vi "Init DAQ.vi"(8 "error in":errorcluster, 11 "Notifiers in":T1) -> (0 "error out":errorcluster, 3 "Notifiers out":T1)   [LabVIEW 2014, in "DAQ.lvlib"]
uses:
  DAQ.lvlib
  support/Message Queue/Message Queue.lvlib
  Support/Message Queue/Enqueue Message (Single).vi
  PLC/PLC.lvlib
  Support/Notifiers/Notifiers.ctl
  Support/Notifiers/Notifiers.lvlib
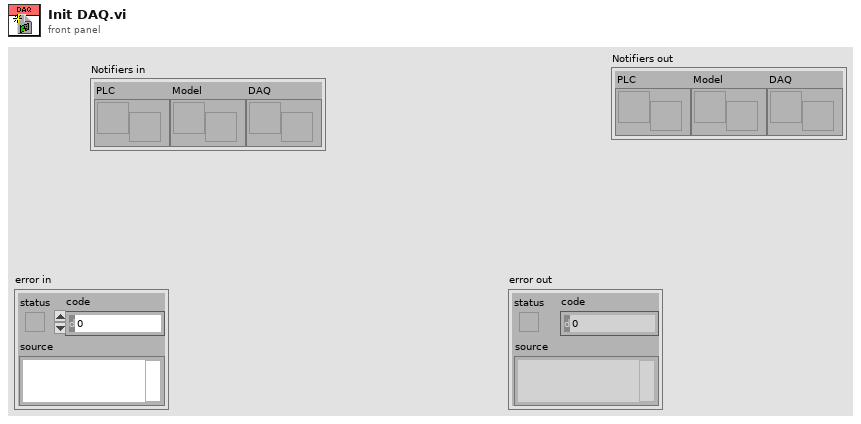
[diagram p1: front panel]
types:
  T1 = typedef "Notifiers.lvlib/Notifiers.ctl" = cluster{"PLC":refnum<notifier>, "Model":refnum<notifier>, "DAQ":refnum<notifier>}
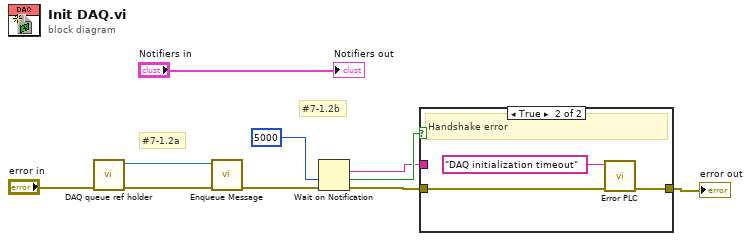
[diagram p0: block diagram]
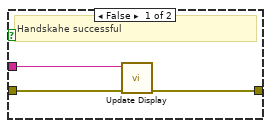
[diagram p2: hidden frame]
diagram:
  # "#7-1.2b"
  # "#7-1.2a"
  n1 = call "DAQ queue ref holder.vi"("error in"="error in") -> ("error out"=w3:errorcluster, "Input Message Queue"=w2:refnum<queue>)  [unwired: 9 in]
  n2 = call-poly "Enqueue Message.vi"("error in (no error)"=w3, "Message Queue"=w2) -> ("error out"=w6:errorcluster)  [unwired: 8 in, 1 out]
  n3 = Wait on Notification(timeout in ms (-1)=5000, error in (no error)=w6) -> (notification=w5:string, timed out?=w8:bool, error out=w9:errorcluster)  [unwired: 2 in, 1 out]
  n4 = case shown="True" w8 {
    tunnel: w9 -> [w12 w15]
    tunnel: [w11 w14] -> w10
    tunnel: w5 -> [w13 _]
    frame False {
      # "Handskahe successful"
      n5 = call "Update Display.vi"("error in"=w12, "Message string"=w13) -> ("error out"=w11:errorcluster)  [unwired: 9 in]
    }
    frame True {
      # "Handshake error"
      n6 = call "Error PLC.vi"("error in"=w15, "String"="DAQ initialization timeout" ("Message")) -> ("error out"=w14:errorcluster)  [unwired: 9 in]
    }
  }
  "error out" <- w10
  "Notifiers out" <- "Notifiers in"
